vi "Recall Hall Effect Results.vi"() -> (2 "Hall Effect Results":T1)   [LabVIEW 2016, in "Hall Effect Library.lvlib"]
uses:
  Hall Effect Library.lvlib
  Private/Global Variables/Hall Effect Data.vi
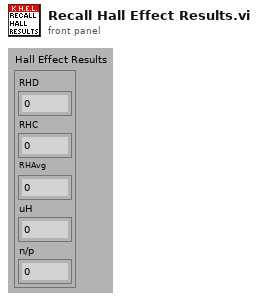
[diagram p1: front panel]
types:
  T1 = cluster{"RHD":dbl, "RHC":dbl, "RHAvg":dbl, "uH":dbl, "n/p":dbl}
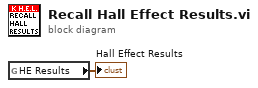
[diagram p0: block diagram]
diagram:
  n1 = global read "Hall Effect Data.vi" "HE Results"() -> (→"Hall Effect Results":T1)
